vi "MEDIDA-IV-BK-8502-ELOAD.vi"() -> ()   [LabVIEW 2013]
doc: "This example shows how to configure a measurement and take multiple readings."
uses:
  <vilib>/Utility/NIReport.llb/HTML Report Image Alignment.ctl
  <vilib>/Utility/NIReport.llb/NI_report.lvclass
  <instrlib>/Keithley 2100 Series/Public/Configure/Configure DC Volts.vi
  <vilib>/Utility/file.llb/Write To Spreadsheet File (DBL).vi
  <vilib>/Utility/NIReport.llb/Append Report Text (str wrap).vi
  <vilib>/Analysis/NI_AALPro.lvlib
  <vilib>/Utility/NIReport.llb/NI_ReportGenerationCore.lvlib
  <instrlib>/Keithley 2100 Series/Keithley 2100 Series.lvlib
  <instrlib>/BK Precision 85XX Series/BK Precision 85XX Series.lvlib
  <instrlib>/Keithley 2100 Series/Public/Configure/Configure AC Volts.vi
  <instrlib>/Keithley 2100 Series/Public/Configure/Configure DC Current.vi
  <instrlib>/Keithley 2100 Series/Public/Configure/Configure 2 Wire Resistance.vi
  <instrlib>/Keithley 2100 Series/Public/Configure/Configure 4 Wire Resistance.vi
  <instrlib>/Keithley 2100 Series/Public/Configure/Configure AC Current.vi
panel:
  in  "Serial Configuration":T1={"Baud Rate"=9600, "Parity"=0, "Data Bits"=8, "Stop Bits"=10} {"Stop Bits" items=["1.0"=10]; "Data Bits" items=["8"=8]; "Parity" items=["None", "Odd", "Even"]; "Baud Rate" items=["4800"=4800, "9600"=9600, "19200"=19200, "38400"=38400]}
  in  "Tab Control 2":enum32{"Page 0", "Page 1", "Page 2"}(tab)
  out "?":dbl[](graph)
  in  "Digital Filter Readings (10)":i32=10
  in  "Digital Filter (0: Off)":u16(ring) items=["Off", "Moving Filter", "Repeating Filter"]
  in  "Delay Time (s)":dbl=1.0
  in  "Salvar em":path
  in  "stop":bool
  out "?":dbl[](graph)
  out "Voltage":dbl
  out "Curva I(V)":cluster{"Y":dbl[], "Y":dbl[]}[](graph)
  out "Fit linear R (Ohms)":dbl format="%#_4p"
  out "Current":dbl format="%#_6e"
  out "Temperatura (ºC)":dbl(slide) scale=0.0..100.0
  in  "Nº de células":dbl=1.0 format="%#.2g"
  out "Efficiency (%)":dbl
  out "Imp (Amps)":dbl
  out "Vmp (Volts)":dbl
  out "Pmax (Watts)":dbl
  out "Rshunt (Ohms)":dbl format="%.5f"
  out "Rseries (Ohms)":dbl format="%.5f"
  out "Fill Factor":dbl format="%.5f"
  out "Voc (Volts)":dbl format="%.5f"
  out "Isc (Amps)":dbl format="%.5f"
  in  "Área total das células (m²)":dbl=0.000988
  out "Luminosidade (W/m²)":dbl(knob) scale=0.0..1500.0
  out "Current and Power vs. Voltage":cluster{"voltage":dbl[], "current":dbl[]}[](graph)=[{"voltage"=[0.00134, 0.011411, 0.025834, 0.043904, 0.055853, 0.075347, 0.099155, 0.125663, 0.165263, 0.217428, 0.267874, 0.315752, 0.36725, 0.425099, 0.474937, 0.530085, 0.588472, 0.643221, 0.694358, 0.754622, 0.812053, 0.873564, 0.938448, 0.995444, 1.055319, 1.116484, 1.181096, 1.242979, 1.310054, 1.384923, 1.457974, 1.528483, 1.591961, 1.655914, 1.723383, 1.78537, 1.841803, 1.874735, 1.918172, 1.968127, 2.017264, 2.064175, 2.116398, 2.158177, 2.191225, 2.218755, 2.24048, 2.261856, 2.280808, 2.297463, 2.312474, 2.325391, 2.338537, 2.350645, 2.362017, 2.372641, 2.381227, 2.390448, 2.39921, 2.407016, 2.414358, 2.421423, 2.428593, 2.435115, 2.441853, 2.447216, 2.45325, 2.459011, 2.464522, 2.470157, 2.474042, 2.47733, 2.481663, 2.486527, 2.491175, 2.496801, 2.501739, 2.507229, 2.511954, 2.515881, 2.519776, 2.523798, 2.526966, 2.530482, 2.534179, 2.537454, 2.540996, 2.544249, 2.547457, 2.550411, 2.553712, 2.556938, 2.559943, 2.562754, 2.565624, 2.568656, 2.571368, 2.573971, 2.576844, 2.579394, 2.581922, 2.584569, 2.58696, 2.589667, 2.592003, 2.594428, 2.596938, 2.59895, 2.601485, 2.603775, 2.606028, 2.608198, 2.610307, 2.6125, 2.614489, 2.616517, 2.618693, 2.620546, 2.622788, 2.624713, 2.626775, 2.628652, 2.630374, 2.632358, 2.634291, 2.635909, 2.637872, 2.639706, 2.6416, 2.64327, 2.64507, 2.646937, 2.64855, 2.650292, 2.651969, 2.653556, 2.655158, 2.656701, 2.658523, 2.66009, 2.661507, 2.663332, 2.664731, 2.666314, 2.667904, 2.669272, 2.67096, 2.672271, 2.67381, 2.675234, 2.676598, 2.67819, 2.679489, 2.681023, 2.682384, 2.683646, 2.68527, 2.686444, 2.688037, 2.689359, 2.69057, 2.692017, 2.693188, 2.694379, 2.695854, 2.697093, 2.698419, 2.699635, 2.700981, 2.702147, 2.703366, 2.704606, 2.705739, 2.707068, 2.708254, 2.70947, 2.710647, 2.711858, 2.713057, 2.714301, 2.71546, 2.716741, 2.717737, 2.719024, 2.720152, 2.72107, 2.722252, 2.723341, 2.724516, 2.725631, 2.726557, 2.727808, 2.728738, 2.72989, 2.731069, 2.732, 2.733089, 2.734104, 2.73519, 2.736257, 2.737217, 2.738296, 2.739307, 2.740423, 2.741454, 2.742348, 2.743357, 2.744268, 2.745417, 2.746408, 2.747273, 2.74838, 2.749326, 2.750382, 2.751351, 2.752211, 2.753257, 2.754209, 2.755152, 2.756018, 2.756854, 2.757837, 2.758826, 2.759727, 2.760683, 2.761421, 2.76238, 2.763236, 2.764109, 2.764945, 2.76579, 2.76688, 2.767667, 2.768646, 2.769522, 2.770365, 2.771362, 2.772145, 2.773009, 2.7739, 2.774781, 2.775641, 2.776447, 2.777355, 2.778196, 2.778952, 2.779808], "current"=[0.11683, 0.116793, 0.116696, 0.116612, 0.116353, 0.116156, 0.115983, 0.115806, 0.115674, 0.115608, 0.115475, 0.115277, 0.115048, 0.114847, 0.114559, 0.114304, 0.114054, 0.113759, 0.113435, 0.11314, 0.112824, 0.112487, 0.112162, 0.111794, 0.111412, 0.111022, 0.11061, 0.110173, 0.109698, 0.109199, 0.108699, 0.1082, 0.107699, 0.107197, 0.106697, 0.106198, 0.105698, 0.105198, 0.104695, 0.104194, 0.103695, 0.103195, 0.102695, 0.102193, 0.101693, 0.101194, 0.100694, 0.10019, 0.09969, 0.09919, 0.098688, 0.098188, 0.097687, 0.097188, 0.096685, 0.096185, 0.095685, 0.095182, 0.094683, 0.094182, 0.093684, 0.093181, 0.092681, 0.09218, 0.091678, 0.091179, 0.090679, 0.090175, 0.089677, 0.089173, 0.088675, 0.088175, 0.087671, 0.087173, 0.086673, 0.086171, 0.085671, 0.085168, 0.08467, 0.08417, 0.083668, 0.083169, 0.082665, 0.082166, 0.081662, 0.081164, 0.080665, 0.080162, 0.079663, 0.079161, 0.07866, 0.078158, 0.077659, 0.077157, 0.076657, 0.076154, 0.075655, 0.075152, 0.074654, 0.074151, 0.073652, 0.07315, 0.07265, 0.072148, 0.071649, 0.071146, 0.070648, 0.070145, 0.069642, 0.069142, 0.068641, 0.068141, 0.067638, 0.067141, 0.066638, 0.066136, 0.065636, 0.065134, 0.064635, 0.064133, 0.063635, 0.063132, 0.062629, 0.06213, 0.061629, 0.061126, 0.060626, 0.060125, 0.059626, 0.059125, 0.058622, 0.058124, 0.057621, 0.057119, 0.056621, 0.056118, 0.055616, 0.055117, 0.054616, 0.054112, 0.053614, 0.053113, 0.05261, 0.052112, 0.051611, 0.051108, 0.05061, 0.050108, 0.049607, 0.049108, 0.048606, 0.048102, 0.047606, 0.047103, 0.046601, 0.046103, 0.045601, 0.045099, 0.044597, 0.044099, 0.043596, 0.043094, 0.042597, 0.042095, 0.041591, 0.041095, 0.040592, 0.040089, 0.039591, 0.03909, 0.038588, 0.038087, 0.037589, 0.037087, 0.036585, 0.036086, 0.035586, 0.035083, 0.034584, 0.034083, 0.033583, 0.033083, 0.032581, 0.03208, 0.031582, 0.03108, 0.030583, 0.030082, 0.029579, 0.02908, 0.02858, 0.028078, 0.02758, 0.02708, 0.026582, 0.026079, 0.025578, 0.025081, 0.02458, 0.02408, 0.02358, 0.023082, 0.02258, 0.022079, 0.021581, 0.021081, 0.020581, 0.020081, 0.019536, 0.019036, 0.018535, 0.018034, 0.017533, 0.017033, 0.016532, 0.016031, 0.01553, 0.01503, 0.014529, 0.014028, 0.013528, 0.013027, 0.012526, 0.012026, 0.011525, 0.011024, 0.010524, 0.010023, 0.009523, 0.009022, 0.008521, 0.00802, 0.007519, 0.007018, 0.006517, 0.006016, 0.005515, 0.005015, 0.004514, 0.004013, 0.003512, 0.003012, 0.002512, 0.002012, 0.001507, 0.001006, 0.000505]}, {"voltage"=[0.00134, 0.011411, 0.025834, 0.043904, 0.055853, 0.075347, 0.099155, 0.125663, 0.165263, 0.217428, 0.267874, 0.315752, 0.36725, 0.425099, 0.474937, 0.530085, 0.588472, 0.643221, 0.694358, 0.754622, 0.812053, 0.873564, 0.938448, 0.995444, 1.055319, 1.116484, 1.181096, 1.242979, 1.310054, 1.384923, 1.457974, 1.528483, 1.591961, 1.655914, 1.723383, 1.78537, 1.841803, 1.874735, 1.918172, 1.968127, 2.017264, 2.064175, 2.116398, 2.158177, 2.191225, 2.218755, 2.24048, 2.261856, 2.280808, 2.297463, 2.312474, 2.325391, 2.338537, 2.350645, 2.362017, 2.372641, 2.381227, 2.390448, 2.39921, 2.407016, 2.414358, 2.421423, 2.428593, 2.435115, 2.441853, 2.447216, 2.45325, 2.459011, 2.464522, 2.470157, 2.474042, 2.47733, 2.481663, 2.486527, 2.491175, 2.496801, 2.501739, 2.507229, 2.511954, 2.515881, 2.519776, 2.523798, 2.526966, 2.530482, 2.534179, 2.537454, 2.540996, 2.544249, 2.547457, 2.550411, 2.553712, 2.556938, 2.559943, 2.562754, 2.565624, 2.568656, 2.571368, 2.573971, 2.576844, 2.579394, 2.581922, 2.584569, 2.58696, 2.589667, 2.592003, 2.594428, 2.596938, 2.59895, 2.601485, 2.603775, 2.606028, 2.608198, 2.610307, 2.6125, 2.614489, 2.616517, 2.618693, 2.620546, 2.622788, 2.624713, 2.626775, 2.628652, 2.630374, 2.632358, 2.634291, 2.635909, 2.637872, 2.639706, 2.6416, 2.64327, 2.64507, 2.646937, 2.64855, 2.650292, 2.651969, 2.653556, 2.655158, 2.656701, 2.658523, 2.66009, 2.661507, 2.663332, 2.664731, 2.666314, 2.667904, 2.669272, 2.67096, 2.672271, 2.67381, 2.675234, 2.676598, 2.67819, 2.679489, 2.681023, 2.682384, 2.683646, 2.68527, 2.686444, 2.688037, 2.689359, 2.69057, 2.692017, 2.693188, 2.694379, 2.695854, 2.697093, 2.698419, 2.699635, 2.700981, 2.702147, 2.703366, 2.704606, 2.705739, 2.707068, 2.708254, 2.70947, 2.710647, 2.711858, 2.713057, 2.714301, 2.71546, 2.716741, 2.717737, 2.719024, 2.720152, 2.72107, 2.722252, 2.723341, 2.724516, 2.725631, 2.726557, 2.727808, 2.728738, 2.72989, 2.731069, 2.732, 2.733089, 2.734104, 2.73519, 2.736257, 2.737217, 2.738296, 2.739307, 2.740423, 2.741454, 2.742348, 2.743357, 2.744268, 2.745417, 2.746408, 2.747273, 2.74838, 2.749326, 2.750382, 2.751351, 2.752211, 2.753257, 2.754209, 2.755152, 2.756018, 2.756854, 2.757837, 2.758826, 2.759727, 2.760683, 2.761421, 2.76238, 2.763236, 2.764109, 2.764945, 2.76579, 2.76688, 2.767667, 2.768646, 2.769522, 2.770365, 2.771362, 2.772145, 2.773009, 2.7739, 2.774781, 2.775641, 2.776447, 2.777355, 2.778196, 2.778952, 2.779808], "current"=[0.0001565522, 0.0013327249229999998, 0.0030147244639999998, 0.0051197332479999995, 0.0064986641089999995, 0.008752006132, 0.011500294365, 0.014552529378000001, 0.019116632262, 0.025136416224, 0.030932750149999997, 0.036398943304, 0.042251378, 0.048821344853, 0.054408307782999994, 0.06059083584, 0.067117585488, 0.073172177739, 0.07876449972999999, 0.08537793308000001, 0.091619067672, 0.098264593668, 0.10525820457599999, 0.111284666536, 0.11757520042799999, 0.123954286648, 0.13064102855999998, 0.136942725367, 0.14371030369200002, 0.151232206677, 0.15848031582600003, 0.1653818606, 0.171452607739, 0.17750901305800001, 0.183879795951, 0.18960272326, 0.194674893494, 0.19721837253, 0.20082301753999998, 0.20506702463799997, 0.20918019047999997, 0.213012539125, 0.21734349260999997, 0.220550582161, 0.22283224392500003, 0.22452469346999998, 0.22560289311999998, 0.22661535264, 0.22737374952, 0.22788535497, 0.22821343411199999, 0.22832549150800002, 0.228444663919, 0.22845448626, 0.22837161364499997, 0.228212474585, 0.22784770549500002, 0.227527621536, 0.22716440043000002, 0.226697580912, 0.226186714872, 0.22563061656299999, 0.22508442783299998, 0.2244689007, 0.22386419933399998, 0.223134707664, 0.22245825675, 0.221741316925, 0.22101093939400002, 0.220271310161, 0.21938567435, 0.21843857275, 0.217569876873, 0.21675801817100002, 0.21591761077500002, 0.215151838971, 0.214326481869, 0.213535679472, 0.21268714517999998, 0.21176170376999998, 0.210824618368, 0.20990175586200002, 0.20889164439, 0.20791958401200003, 0.20694612549799998, 0.205949916456, 0.20496944233999997, 0.20395208833800002, 0.202938066991, 0.201893085171, 0.20087498591999997, 0.19984516020400003, 0.198802613437, 0.19773441037800002, 0.196673038968, 0.19561342902399997, 0.19453684604000002, 0.19343906859199997, 0.19237171197599998, 0.191264644494, 0.190163719144, 0.18906122235000003, 0.18794264400000002, 0.186839294716, 0.18571442294700002, 0.18458317448800002, 0.18346847582400003, 0.18230334774999998, 0.18117261836999998, 0.18003021105, 0.17888036794799997, 0.17772521991799997, 0.17655594486600001, 0.1754058625, 0.174224317982, 0.173045968312, 0.171880533748, 0.170686643164, 0.16952390237999998, 0.16833071882899997, 0.167154827125, 0.16595205806399999, 0.16473769324600002, 0.16354840254, 0.16234872003900003, 0.161122573534, 0.159923627872, 0.15871232324999998, 0.15750804159999998, 0.15628333874999997, 0.15505929354, 0.153850566188, 0.15261209955000002, 0.151382028748, 0.15015713674899997, 0.148912255608, 0.147669267328, 0.146429389017, 0.145197892168, 0.14394279008, 0.142694036298, 0.141457552516, 0.14019149791, 0.13894695516799999, 0.137693193344, 0.136421153376, 0.1351772856, 0.13390215526799998, 0.13263969267, 0.131375391272, 0.130098722388, 0.12882629537999998, 0.127559753334, 0.126284226369, 0.12500177678399998, 0.12372413153799999, 0.12245099727000001, 0.12115593795599999, 0.11987838608899999, 0.118598042541, 0.11729808972000001, 0.11600978059799999, 0.11472172923600002, 0.113419884005, 0.11212326371400001, 0.110837036835, 0.109534224048, 0.10822566751499998, 0.10693453877100001, 0.10562692623, 0.10431748720799999, 0.10301032872200001, 0.10170602327099999, 0.10039703091600001, 0.09908147259000001, 0.09777393442, 0.096461084142, 0.09514011421400001, 0.093828363288, 0.092511520983, 0.09119329318000001, 0.089877942503, 0.088546589197, 0.08722628991999999, 0.085907840464, 0.08457085560000001, 0.08325463291600001, 0.08192354396200001, 0.080588458764, 0.07926134948, 0.07792499906000001, 0.07659139302399999, 0.07525859404, 0.07392542120000001, 0.072597276158, 0.07124782800000001, 0.069906950442, 0.06857406242399999, 0.0672309702, 0.06588906856, 0.06454357686, 0.063205348272, 0.061853552060000004, 0.060505799417, 0.059163318774, 0.05781143818799999, 0.056461030417, 0.055107645708, 0.05363446651200001, 0.052280622688, 0.050920705054999994, 0.04956428492000001, 0.048203932758, 0.046847256606, 0.045485334732000005, 0.044120694541, 0.04275808121, 0.04139576127, 0.040029603408, 0.038661420504, 0.037294720912, 0.035926342599, 0.034557054476, 0.033188476902, 0.031816871575, 0.030441905104, 0.02907128712, 0.027695914428000002, 0.026322610007, 0.024945333790000003, 0.02356729659, 0.0221903776, 0.020810088172999997, 0.019430357627999998, 0.018048974874, 0.01666651584, 0.015284061429999999, 0.013902307175000002, 0.012517362625999999, 0.011131660699999999, 0.009745030872, 0.008360230691999999, 0.006974434864, 0.00558803826, 0.004186741372, 0.0027956257119999997, 0.0014038030400000002]}]
  in  "Tab Control":enum32{"INICIAL", "CONFIG"}(tab)=enum."CONFIG"
  in  "BK 8500":refnum<visa-resource-name>="GPIB0::24::INSTR"
  in  "Keithley 2100 Pyranometer":refnum<visa-resource-name>="GPIB::16"
  in  "Keithley 2100 PT100":refnum<visa-resource-name>="GPIB::16"
  in  "Monitorar?":bool
  in  "Multimetro p/ V":refnum<visa-resource-name>
  in  "Salvar Medidas em":path
  in  "Fonte Inicial (V ou A)":dbl format="%.3e"
  in  "Fonte Final (V ou A)":dbl format="%.3e"
  in  "Passo Fonte (V ou A)":dbl format="%.3e"
  in  "Salvar relatório em":path
  in  "Maximum Input Voltage (0)":dbl min=0.0 max=120.0 format="%#_3g"
  in  "Maximum Input Current (0)":dbl min=0.0 max=30.0 format="%#_3g"
  in  "Maximum Input Power (0)":dbl min=0.0 max=300.0 step=1.0 format="%#_3g"
  # "Programa desenvolvido \nem plataforma LABVIEW 2010:\n2017\nLSD/UNIFEI\nRero e Davi"
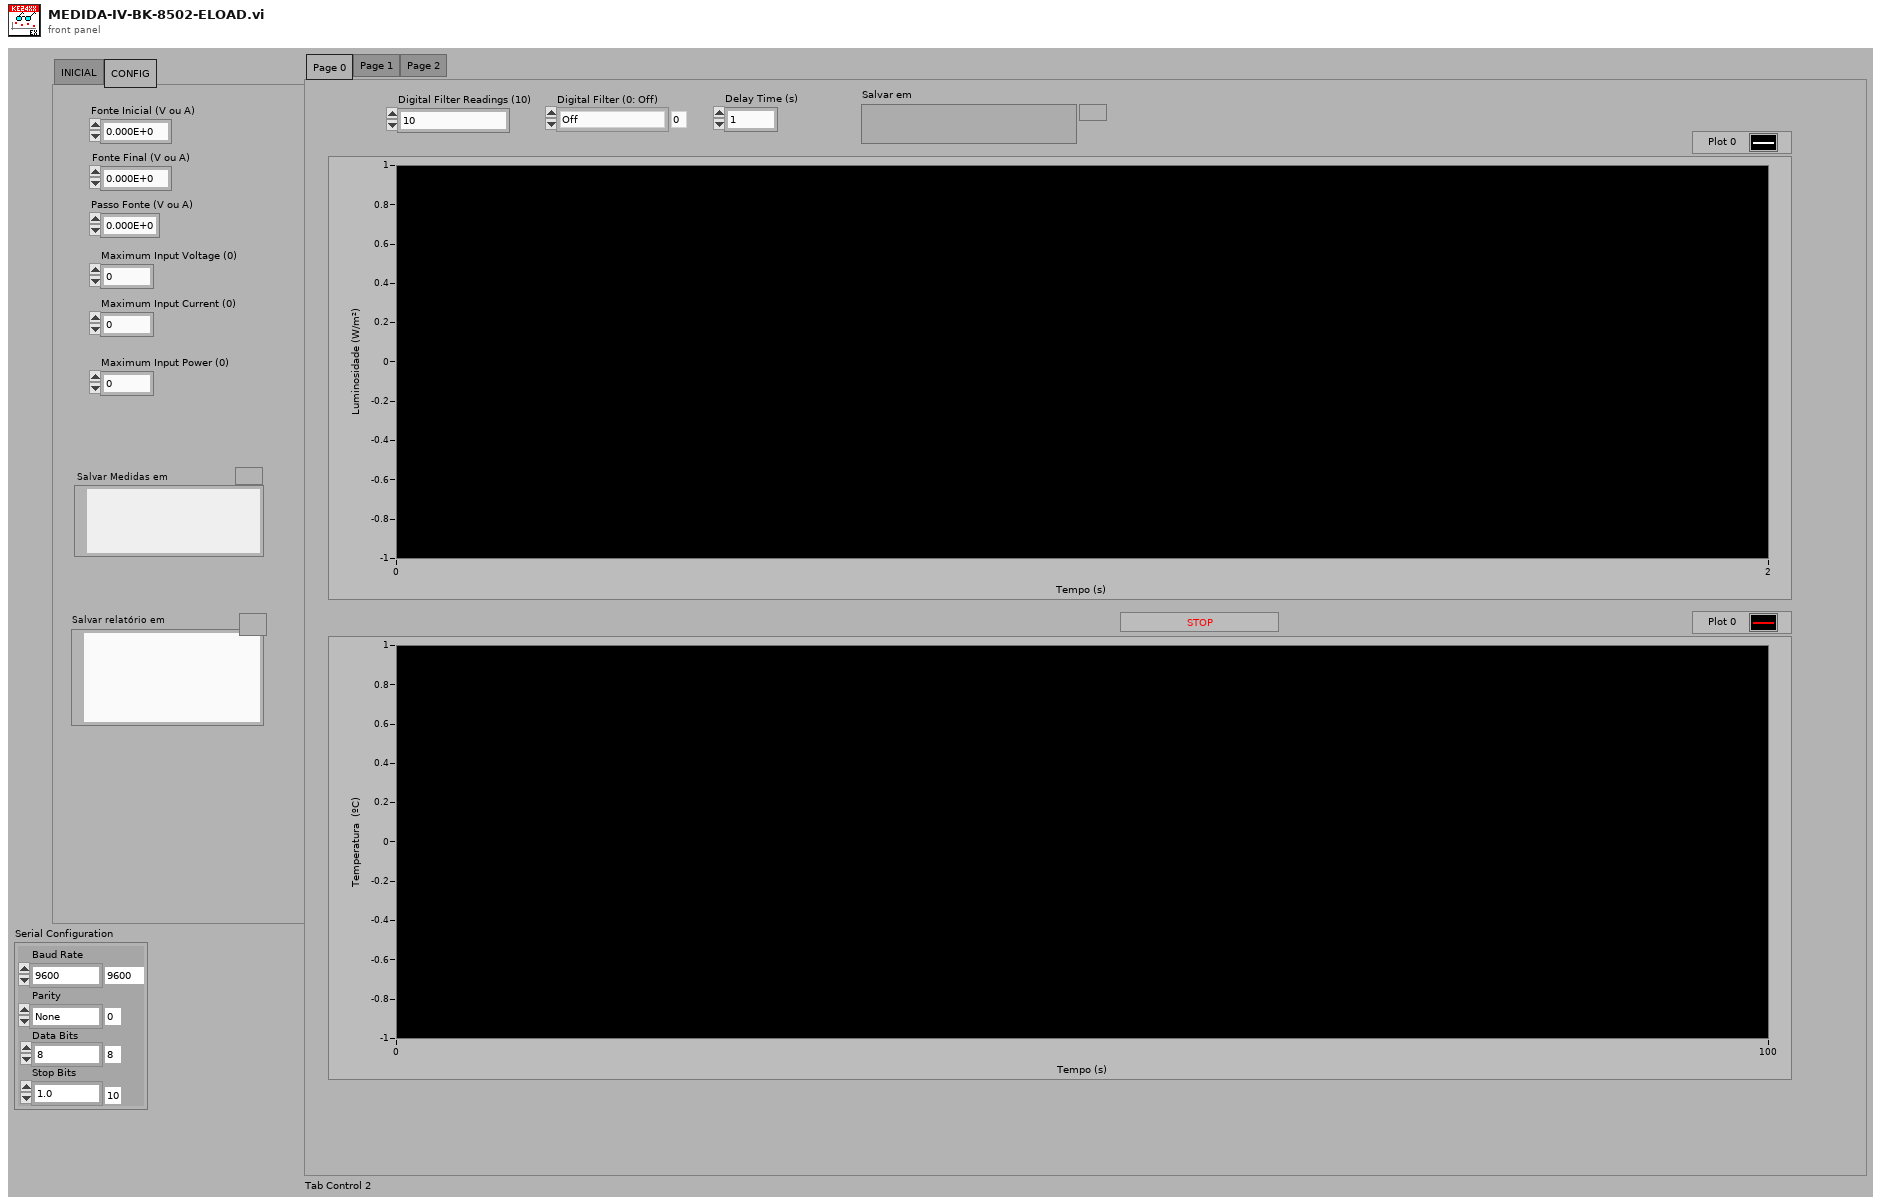
[diagram p1: front panel]
types:
  T1 = cluster{"Baud Rate":u32, "Parity":u16, "Data Bits":u16, "Stop Bits":u16}
  T2 = typedef "NI_ReportGenerationCore.lvlib/HTML Report Image Alignment.ctl" = enum16{"(default)", "LEFT", "RIGHT", "TOP", "TEXTTOP", "MIDDLE", "ABSMIDDLE", "BASELINE", "BOTTOM", "ABSBOTTOM"}
  T3 = cluster{"Italic":enum16{"Italic Unchanged", "Italic On", "Italic Off"}, "Strike Through":enum16{"Strike Through Unchanged", "Strike Through On", "Strike Through Off"}, "Underline":enum16{"Underline Unchanged", "Underline On", "Underline Off"}, "Bold":enum16{"Bold Unchanged", "Bold On", "Bold Off"}}
  T4 = enum16{"Standard Report", "HTML", "Word", "Excel"}
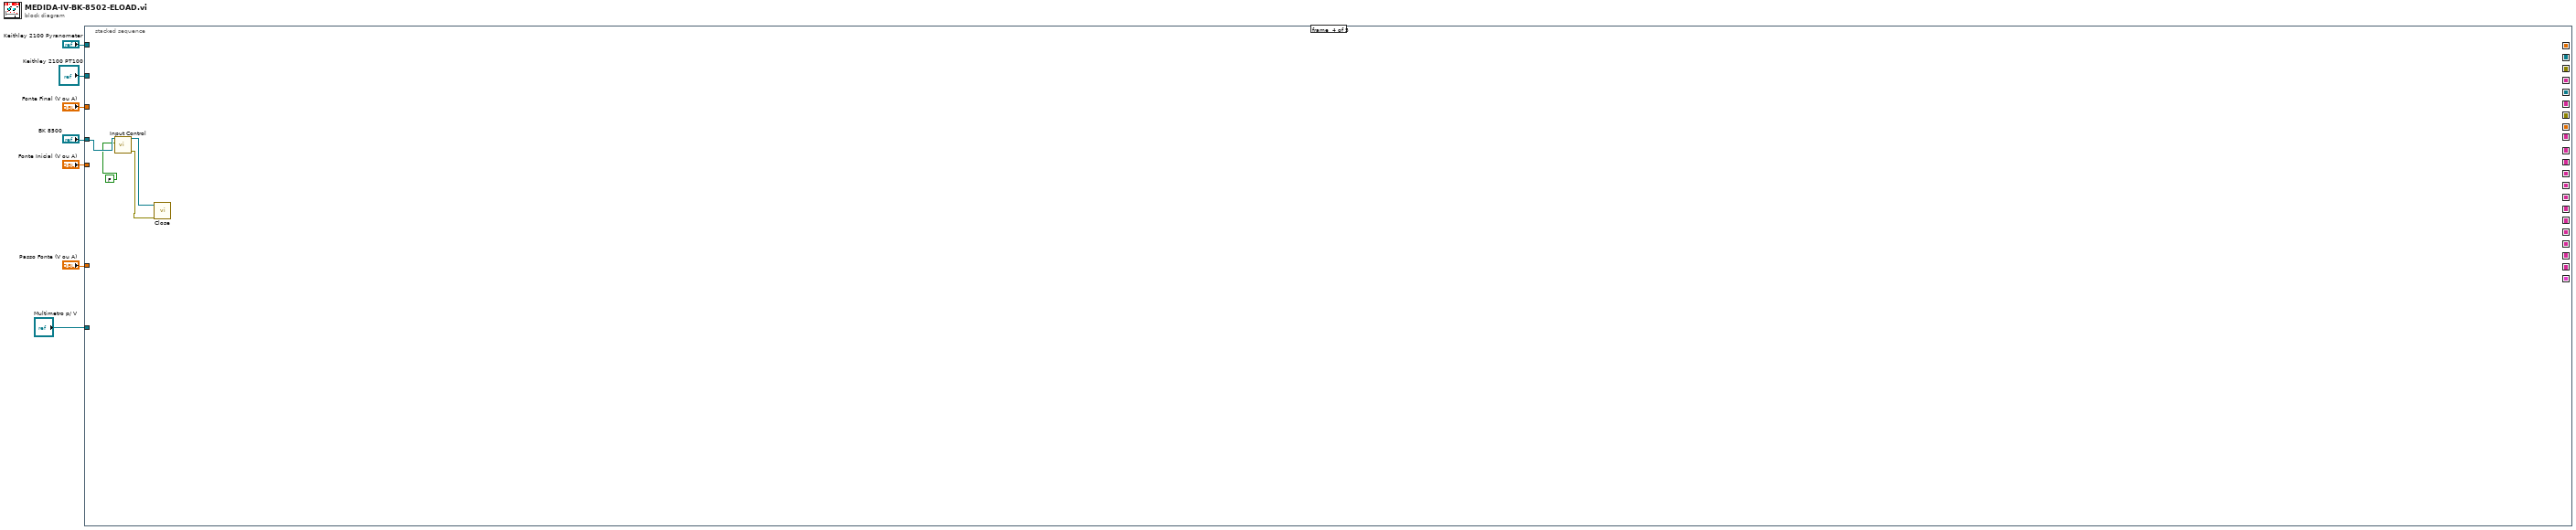
[diagram p0: block diagram]
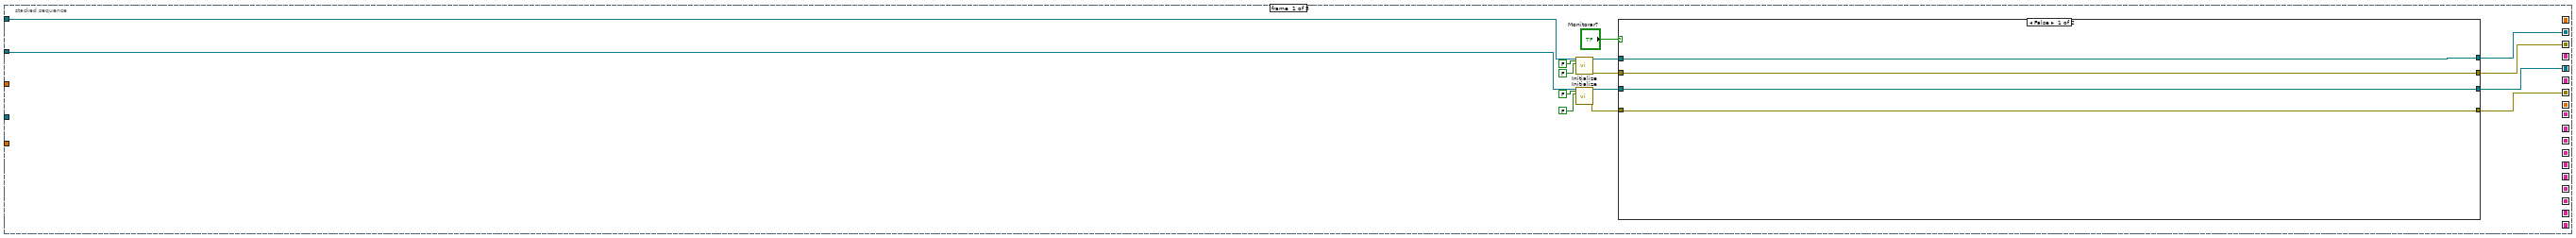
[diagram p2: hidden frame]
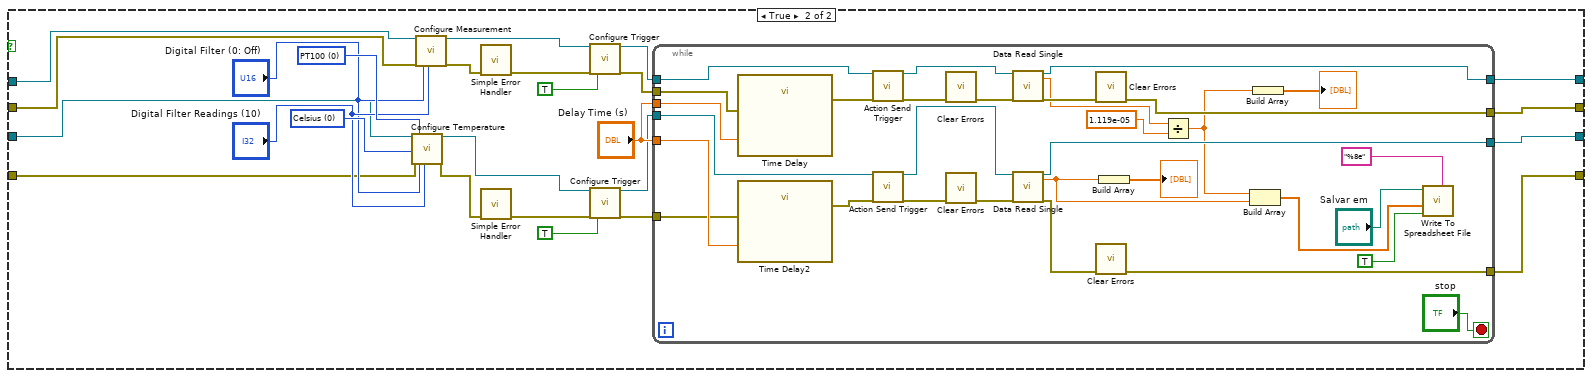
[diagram p3: hidden frame]
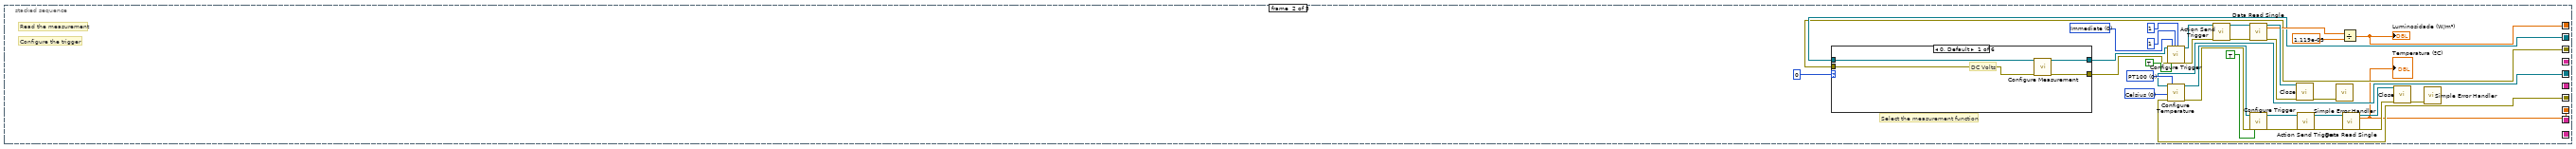
[diagram p4: hidden frame]
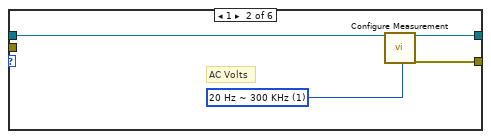
[diagram p5: hidden frame]
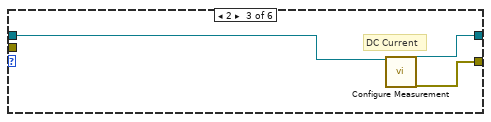
[diagram p6: hidden frame]
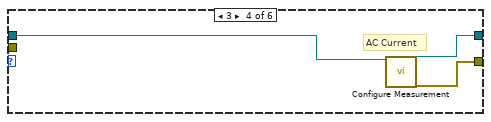
[diagram p7: hidden frame]
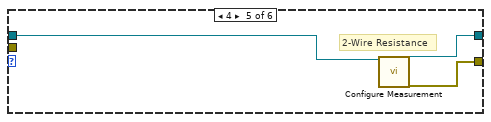
[diagram p8: hidden frame]
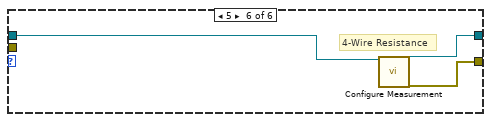
[diagram p9: hidden frame]
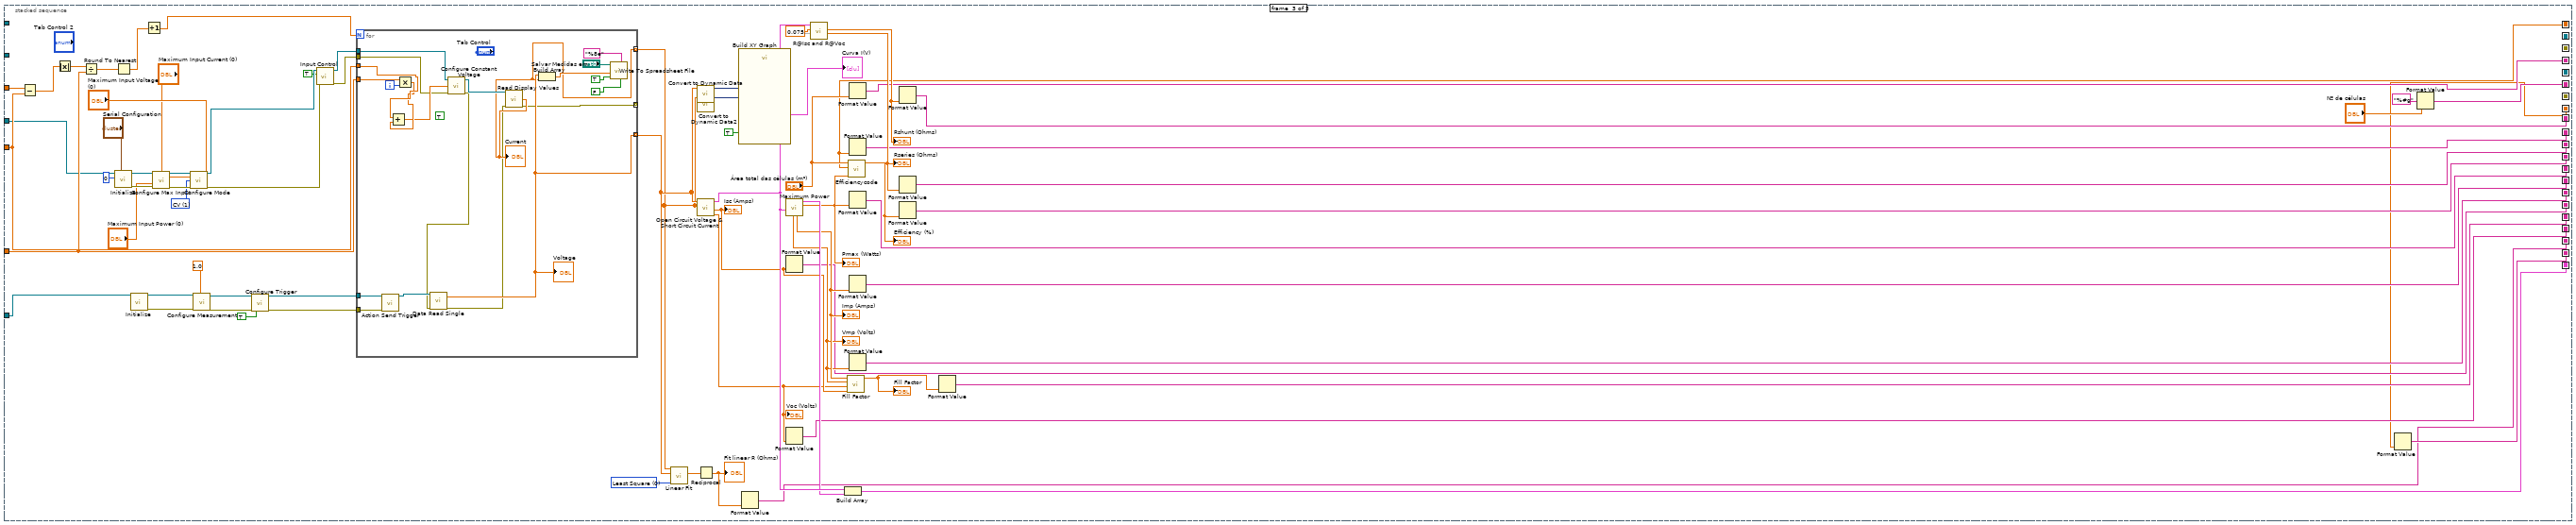
[diagram p10: hidden frame]
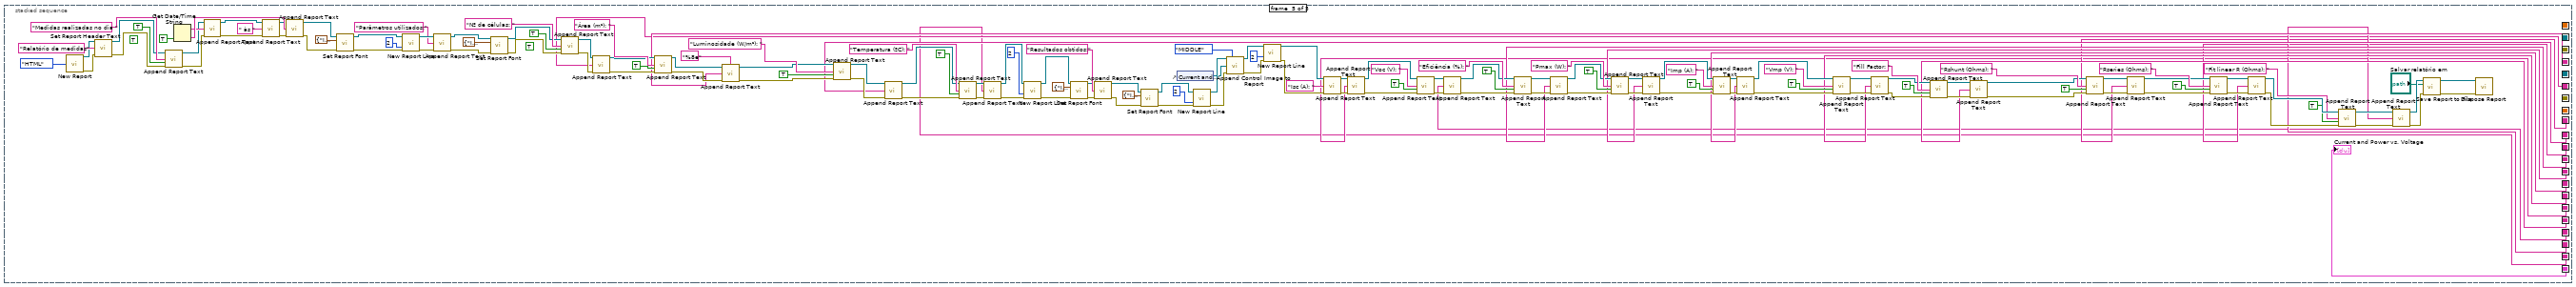
[diagram p11: hidden frame]
diagram:
  n1 = stacked-sequence {
    seq-local: [_ w100 _ _ _] -> [_ _ w180 _ _]
    seq-local: [_ _ w179 _ _] -> [_ _ _ _ w239]
    seq-local: [_ _ w178 _ _] -> [_ _ _ _ w240]
    seq-local: [_ _ w177 _ _] -> [_ _ _ _ w241]
    seq-local: [_ _ w176 _ _] -> [_ _ _ _ w242]
    seq-local: [_ _ w175 _ _] -> [_ _ _ _ w243]
    seq-local: [_ _ w174 _ _] -> [_ _ _ _ w244]
    seq-local: [_ _ w173 _ _] -> [_ _ _ _ w246]
    seq-local: [_ _ w172 _ _] -> [_ _ _ _ w247]
    seq-local: [_ _ w171 _ _] -> [_ _ _ _ w248]
    seq-local: [_ _ w170 _ _] -> [_ _ _ _ w249]
    seq-local: [_ _ w169 _ _] -> [_ _ _ _ w250]
    seq-local: [_ _ w168 _ _] -> [_ _ _ _ w251]
    seq-local: [_ _ w167 _ _] -> [_ _ _ _ w252]
    seq-local: [_ _ w166 _ _] -> [_ _ _ _ w245]
    seq-local: [_ _ w165 _ _] -> [_ _ _ _ w238]
    seq-local: [_ w83 _ _ _] -> [_ _ w163 _ _]
    seq-local: [w19 _ _ _ _] -> [_ w93 _ _ _]
    seq-local: [w20 _ _ _ _] -> [_ w94 _ _ _]
    seq-local: [w18 _ _ _ _] -> [_ w92 _ _ _]
    seq-local: [w17 _ _ _ _] -> [_ w91 _ _ _]
    tunnel: "BK 8500" -> [_ _ w152 w235 _]
    tunnel: "Fonte Inicial (V ou A)" -> [_ _ w205 _ _]
    tunnel: "Fonte Final (V ou A)" -> [_ _ w204 _ _]
    tunnel: "Passo Fonte (V ou A)" -> [_ _ w203 _ _]
    tunnel: "Keithley 2100 Pyranometer" -> [w22 _ _ _ _]
    tunnel: "Keithley 2100 PT100" -> [w21 _ _ _ _]
    tunnel: "Multimetro p/ V" -> [_ _ w155 _ _]
    frame #0 {
      n2 = call <instrlib>:"Initialize.vi"("VISA resource name"=w22, "ID Query? (T: Check)"=FALSE, "Reset? (T: Reset)"=FALSE) -> ("VISA resource name out"=w10:refnum<visa-resource-name>, "error out"=w9:errorcluster)  [unwired: 15 in]
      n3 = call <instrlib>:"Initialize.vi"("VISA resource name"=w21, "ID Query? (T: Check)"=FALSE, "Reset? (T: Reset)"=FALSE) -> ("VISA resource name out"=w12:refnum<visa-resource-name>, "error out"=w11:errorcluster)  [unwired: 15 in]
      n4 = case shown="False" "Monitorar?" {
        tunnel: [w26 w44] -> w20
        tunnel: [w24 w28] -> w19
        tunnel: [w25 w43] -> w18
        tunnel: [w23 w27] -> w17
        tunnel: w12 -> [w24 w35]
        tunnel: w11 -> [w23 w34]
        tunnel: w10 -> [w26 w33]
        tunnel: w9 -> [w25 w32]
        frame False {
        }
        frame True {
          w38 = u16 0 items=["PT100", "D100", "F100", "PT385", "PT3916", "User-Defined", "SPRTD", "NTCT"] ("RTD Type  (PT100)")
          w47 = u16 0 items=["Celsius", "Fahrenheit", "Kelvin"] ("Temperature Units (0: Celsius)")
          n5 = call <instrlib>:"Configure Temperature.vi"("VISA resource name"=w35, "Temperature Units (0: Celsius)"=w47, "error in (no error)"=w34, "RTD Type  (PT100)"=w38, "Digital Filter (0: Off)"="Digital Filter (0: Off)", "Digital Filter Readings (10)"="Digital Filter Readings (10)") -> ("VISA resource name out"=w46:refnum<visa-resource-name>, "error out"=w40:errorcluster)  [unwired: 12 in]
          n6 = call-poly <instrlib>:"Configure Measurement.vi"("VISA resource name"=w33, "error in (no error)"=w32, "Digital Filter (0: Off)"="Digital Filter (0: Off)", "Digital Filter Readings (10)"="Digital Filter Readings (10)") -> ("VISA resource name out"=w50:refnum<visa-resource-name>, "error out"=w42:errorcluster)  [unwired: 14 in]
          n7 = call <vilib>:"Simple Error Handler.vi"("error in (no error)"=w42) -> ("error out"=w41:errorcluster)  [unwired: 4 in, 4 out]
          n8 = call <vilib>:"Simple Error Handler.vi"("error in (no error)"=w40) -> ("error out"=w39:errorcluster)  [unwired: 4 in, 4 out]
          n9 = call <instrlib>:"Configure Trigger.vi"("VISA resource name"=w50, "error in (no error)"=w41, "Auto Delay? (T: Auto)"=TRUE) -> ("VISA resource name out"=w48:refnum<visa-resource-name>, "error out"=w49:errorcluster)  [unwired: 15 in]
          n10 = call <instrlib>:"Configure Trigger.vi"("VISA resource name"=w46, "error in (no error)"=w39, "Auto Delay? (T: Auto)"=TRUE) -> ("VISA resource name out"=w30:refnum<visa-resource-name>, "error out"=w29:errorcluster)  [unwired: 15 in]
          n11 = while {
            tunnel: w49 -> [w80]
            tunnel: "Delay Time (s)" -> [w79]
            tunnel: w48 -> [w77]
            tunnel: [w70] -> w43
            tunnel: [w73] -> w44
            tunnel: "Delay Time (s)" -> [w60]
            tunnel: w30 -> [w59]
            tunnel: w29 -> [w58]
            tunnel: [w57] -> w28
            tunnel: [w56] -> w27
            stop <- "stop" stop-if-true
            n12 = call "Time Delay"("error in (no error)"=w80, "Delay Time (s)"=w79) -> ("error out"=w78:errorcluster)  [unwired: 9 in]
            n13 = call "Time Delay2"("error in (no error)"=w58, "Delay Time (s)"=w60) -> ("error out"=w66:errorcluster)  [unwired: 9 in]
            n14 = call <instrlib>:"Action Send Trigger.vi"("VISA resource name"=w77, "error in (no error)"=w78) -> ("VISA resource name out"=w82:refnum<visa-resource-name>, "error out"=w69:errorcluster)  [unwired: 16 in]
            n15 = call <instrlib>:"Action Send Trigger.vi"("VISA resource name"=w59, "error in (no error)"=w66) -> ("VISA resource name out"=w65:refnum<visa-resource-name>, "error out"=w64:errorcluster)  [unwired: 16 in]
            n16 = call <vilib>:"Clear Errors.vi"("error in (no error)"=w69) -> ("error out"=w68:errorcluster)  [unwired: 6 in]
            n17 = call <vilib>:"Clear Errors.vi"("error in (no error)"=w64) -> ("error out"=w63:errorcluster)  [unwired: 6 in]
            n18 = call <instrlib>:"Data Read Single.vi"("VISA resource name"=w82, "error in (no error)"=w68) -> ("VISA resource name out"=w73:refnum<visa-resource-name>, "Measurement"=w55:dbl, "error out"=w71:errorcluster)  [unwired: 15 in]
            n19 = call <instrlib>:"Data Read Single.vi"("VISA resource name"=w65, "error in (no error)"=w63) -> ("VISA resource name out"=w57:refnum<visa-resource-name>, "Measurement"=w53:dbl, "error out"=w62:errorcluster)  [unwired: 15 in]
            n20 = call <vilib>:"Clear Errors.vi"("error in (no error)"=w71) -> ("error out"=w70:errorcluster)  [unwired: 6 in]
            n21 = call <vilib>:"Clear Errors.vi"("error in (no error)"=w62) -> ("error out"=w56:errorcluster)  [unwired: 6 in]
            n22 = Build Array(w53) -> (→"?":dbl[])
            n23 = Divide(x=w55, y=1.119e-05) -> (x/y=w54:dbl)
            n24 = Build Array(w54, w53) -> (w52:dbl[])
            n25 = Build Array(w54) -> (→"?":dbl[])
            n26 = call-poly <vilib>:"Write To Spreadsheet File.vi"("format (%.3f)"="%8e", "append to file? (new file:F)"=TRUE, "1D data"=w52, "file path (dialog if empty)"="Salvar em") -> ()  [unwired: 4 in, 1 out]
          }
        }
      }
    }
    frame #1 {
      w95 = u16 0 items=["PT100", "D100", "F100", "PT385", "PT3916", "User-Defined", "SPRTD", "NTCT"] ("RTD Type  (PT100)")
      w96 = u16 0 items=["Celsius", "Fahrenheit", "Kelvin"] ("Temperature Units (0: Celsius)")
      w113 = u16 0 items=["Immediate", "Bus", "External"] ("Source (0: Immediate)")
      # "Read the measurement"
      # "Configure the trigger"
      # "Select the measurement function"
      n27 = case shown="0, Default" u16 0 ("Function (0: DC Volts)") {
        tunnel: w94 -> [w120 w124 w127 w130 w133 w136]
        tunnel: [w119 w123 w126 w129 w132 w135] -> w109
        tunnel: [w118 w122 w125 w128 w131 w134] -> w110
        tunnel: w92 -> [w117 _ _ _ _ _]
        frame 0, Default {
          # "DC Volts"
          n28 = call-poly <instrlib>:"Configure Measurement.vi"("VISA resource name"=w120, "error in (no error)"=w117) -> ("VISA resource name out"=w118:refnum<visa-resource-name>, "error out"=w119:errorcluster)  [unwired: 16 in]
        }
        frame 1 {
          w121 = u16 1 items=["3 Hz ~ 300 KHz", "20 Hz ~ 300 KHz", "200 Hz ~ 300 KHz"] ("Bandwidth (20 Hz)")
          # "AC Volts"
          n29 = call-poly <instrlib>:"Configure Measurement.vi"("VISA resource name"=w124, "Bandwidth (20 Hz)"=w121) -> ("VISA resource name out"=w122:refnum<visa-resource-name>, "error out"=w123:errorcluster)  [unwired: 16 in]
        }
        frame 2 {
          # "DC Current"
          n30 = call-poly <instrlib>:"Configure Measurement.vi"("VISA resource name"=w127) -> ("VISA resource name out"=w125:refnum<visa-resource-name>, "error out"=w126:errorcluster)  [unwired: 17 in]
        }
        frame 3 {
          # "AC Current"
          n31 = call-poly <instrlib>:"Configure Measurement.vi"("VISA resource name"=w130) -> ("VISA resource name out"=w128:refnum<visa-resource-name>, "error out"=w129:errorcluster)  [unwired: 17 in]
        }
        frame 4 {
          # "2-Wire Resistance"
          n32 = call-poly <instrlib>:"Configure Measurement.vi"("VISA resource name"=w133) -> ("VISA resource name out"=w131:refnum<visa-resource-name>, "error out"=w132:errorcluster)  [unwired: 17 in]
        }
        frame 5 {
          # "4-Wire Resistance"
          n33 = call-poly <instrlib>:"Configure Measurement.vi"("VISA resource name"=w136) -> ("VISA resource name out"=w134:refnum<visa-resource-name>, "error out"=w135:errorcluster)  [unwired: 17 in]
        }
      }
      n34 = call <instrlib>:"Configure Trigger.vi"("VISA resource name"=w110, "error in (no error)"=w109, "Source (0: Immediate)"=w113, "Auto Delay? (T: Auto)"=TRUE, "Sample Count (1)"=1, "Trigger Count (1)"=1) -> ("VISA resource name out"=w105:refnum<visa-resource-name>, "error out"=w104:errorcluster)  [unwired: 12 in]
      n35 = call <instrlib>:"Configure Temperature.vi"("VISA resource name"=w93, "Temperature Units (0: Celsius)"=w96, "error in (no error)"=w91, "RTD Type  (PT100)"=w95) -> ("VISA resource name out"=w90:refnum<visa-resource-name>, "error out"=w89:errorcluster)  [unwired: 14 in]
      n36 = call <instrlib>:"Action Send Trigger.vi"("VISA resource name"=w105, "error in (no error)"=w104) -> ("VISA resource name out"=w112:refnum<visa-resource-name>, "error out"=w111:errorcluster)  [unwired: 16 in]
      n37 = call <instrlib>:"Data Read Single.vi"("VISA resource name"=w112, "error in (no error)"=w111) -> ("VISA resource name out"=w107:refnum<visa-resource-name>, "Measurement"=w101:dbl, "error out"=w106:errorcluster)  [unwired: 15 in]
      n38 = call <instrlib>:"Configure Trigger.vi"("VISA resource name"=w90, "error in (no error)"=w89, "Auto Delay? (T: Auto)"=TRUE) -> ("VISA resource name out"=w87:refnum<visa-resource-name>, "error out"=w86:errorcluster)  [unwired: 15 in]
      n39 = call <instrlib>:"Close.vi"("VISA resource name"=w107, "error in (no error)"=w106) -> ("error out"=w108:errorcluster)  [unwired: 17 in]
      n40 = call <instrlib>:"Action Send Trigger.vi"("VISA resource name"=w87, "error in (no error)"=w86) -> ("VISA resource name out"=w85:refnum<visa-resource-name>, "error out"=w84:errorcluster)  [unwired: 16 in]
      n41 = call <vilib>:"Simple Error Handler.vi"("error in (no error)"=w108) -> ()  [unwired: 4 in, 5 out]
      n42 = Divide(x=w101, y=1.119e-05) -> (x/y=w100:dbl)
      "Luminosidade (W/m²)" <- w100
      n43 = call <instrlib>:"Data Read Single.vi"("VISA resource name"=w85, "error in (no error)"=w84) -> ("VISA resource name out"=w98:refnum<visa-resource-name>, "Measurement"=w83:dbl, "error out"=w97:errorcluster)  [unwired: 15 in]
      "Temperatura (ºC)" <- w83
      n44 = call <instrlib>:"Close.vi"("VISA resource name"=w98, "error in (no error)"=w97) -> ("error out"=w99:errorcluster)  [unwired: 17 in]
      n45 = call <vilib>:"Simple Error Handler.vi"("error in (no error)"=w99) -> ()  [unwired: 4 in, 5 out]
    }
    frame #2 {
      w145 = u16 1 items=["CC", "CV", "CW", "CR"] ("Mode of Operation (0:CC)")
      w198 = u16 0 items=["Least Square", "Least Absolute Residual", "Bisquare"] ("method")
      n46 = Subtract(x=w204, y=w205) -> (x-y=w210:dbl)
      n47 = Absolute Value(x=w210) -> (abs(x)=w209:dbl)
      n48 = Divide(x=w209, y=w203) -> (x/y=w208:dbl)
      n49 = call <instrlib>:"Initialize.vi"("Serial Configuration"="Serial Configuration", "Communication Address (0)"=u8 0, "VISA resource name"=w152) -> ("error out"=w148:errorcluster, "VISA resource name out"=w149:refnum<visa-resource-name>)  [unwired: 7 in]
      n50 = Round To Nearest(number=w208) -> (nearest integer value=w207:dbl)
      n51 = call <instrlib>:"Initialize.vi"("VISA resource name"=w155) -> ("VISA resource name out"=w154:refnum<visa-resource-name>, "error out"=w153:errorcluster)  [unwired: 17 in]
      n52 = Increment(x=w207) -> (x+1=w206:dbl)
      n53 = call <instrlib>:"Configure Max Input.vi"("VISA resource name"=w149, "Maximum Input Voltage (0)"="Maximum Input Voltage (0)", "Maximum Input Current (0)"="Maximum Input Current (0)", "Maximum Input Power (0)"="Maximum Input Power (0)", "error in (no error)"=w148) -> ("VISA resource name out"=w147:refnum<visa-resource-name>, "error out"=w146:errorcluster)  [unwired: 9 in]
      n54 = call <instrlib>:"Configure Mode.vi"("VISA resource name"=w147, "Mode of Operation (0:CC)"=w145, "error in (no error)"=w146) -> ("VISA resource name out"=w144:refnum<visa-resource-name>, "error out"=w139:errorcluster)  [unwired: 11 in]
      n55 = call-poly <instrlib>:"Configure Measurement.vi"("VISA resource name"=w154, "error in (no error)"=w153, "Custom Range (100mV)"=1.0) -> ("VISA resource name out"=w162:refnum<visa-resource-name>, "error out"=w161:errorcluster)  [unwired: 15 in]
      n56 = call <instrlib>:"Configure Trigger.vi"("VISA resource name"=w162, "error in (no error)"=w161, "Auto Delay? (T: Auto)"=TRUE) -> ("VISA resource name out"=w159:refnum<visa-resource-name>, "error out"=w158:errorcluster)  [unwired: 15 in]
      n57 = call <instrlib>:"Input Control.vi"("error in (no error)"=w139, "Enable Input Terminals (F: Off)"=TRUE, "VISA resource name"=w144) -> ("error out"=w138:errorcluster, "VISA resource name out"=w143:refnum<visa-resource-name>)  [unwired: 7 in]
      n58 = for {
        N: w206 -> [_]
        tunnel: w205 -> [w219]
        tunnel: w203 -> [w227]
        tunnel: [w221] -> w193 mode=indexing
        tunnel: [w215] -> w157 mode=indexing
        tunnel: w159 -> [w224]
        tunnel: w158 -> [w223]
        tunnel: [w211] -> _ mode=indexing
        tunnel: w143 -> [w220]
        tunnel: w138 -> [w214]
        i -> [w226]
        (unwired) TRUE ("Enable Output (T: Enable)")
        n59 = call <instrlib>:"Action Send Trigger.vi"("VISA resource name"=w224, "error in (no error)"=w223) -> ("VISA resource name out"=w222:refnum<visa-resource-name>)  [unwired: 16 in, 1 out]
        n60 = Multiply(x=w227, y=w226) -> (x*y=w218:dbl)
        n61 = Add(x=w219, y=w218) -> (x+y=w217:dbl)
        n62 = call <instrlib>:"Configure Constant Voltage.vi"("VISA resource name"=w220, "CV Voltage (0)"=w217, "error in (no error)"=w214) -> ("VISA resource name out"=w216:refnum<visa-resource-name>, "error out"=w213:errorcluster)  [unwired: 11 in]
        n63 = call <instrlib>:"Data Read Single.vi"("VISA resource name"=w222, "error in (no error)"=w213) -> ("Measurement"=w221:dbl, "error out"=w212:errorcluster)  [unwired: 15 in, 1 out]
        "Voltage" <- w221
        n64 = call <instrlib>:"Read Display Values.vi"("VISA resource name"=w216, "error in (no error)"=w212) -> ("Terminal Input Current (A)"=w215:dbl, "error out"=w211:errorcluster)  [unwired: 9 in, 3 out]
        "Current" <- w215
        n65 = Build Array(w221, w215) -> (w225:dbl[])
        n66 = call-poly <vilib>:"Write To Spreadsheet File.vi"("transpose? (no:F)"=FALSE ("append to file? (new file:F)"), "format (%.3f)"="%8e", "append to file? (new file:F)"=TRUE, "1D data"=w225, "file path (dialog if empty)"="Salvar Medidas em") -> ()  [unwired: 3 in, 1 out]
      }
      n67 = call <vilib>:"Linear Fit.vi"("Y"=w157, "X"=w193, "method"=w198) -> ("slope"=w197:dbl)  [unwired: 8 in, 4 out]
      n68 = call "Convert to Dynamic Data"("Array"=w193) -> ("Dynamic Data Type"=w200:dynamicdata)  [unwired: 3 in]
      n69 = call "Convert to Dynamic Data2"("Array"=w157) -> ("Dynamic Data Type"=w199:dynamicdata)  [unwired: 3 in]
      n70 = call "Open Circuit Voltage & Short Circuit Current.vi"("current"=w157, "voltage"=w193) -> ("open circuit voltage"=w189:dbl, "short circuit current"=w190:dbl, "Current (Amps) vs Voltage (Volts)"=w195:cluster{"voltage":dbl[], "current":dbl[]})  [unwired: 7 out]
      "Voc (Volts)" <- w189
      "Isc (Amps)" <- w190
      n71 = Reciprocal(x=w197) -> (1/x=w181:dbl)
      "Fit linear R (Ohms)" <- w181
      n72 = call "Build XY Graph"("Reset"=TRUE, "Y Input"=w199, "X Input"=w200) -> ("XY Graph"=→"Curva I(V)":cluster{"Y":dbl[], "Y":dbl[]}[])  [unwired: 7 in, 1 out]
      n73 = Format Value(value (0)=w181) -> (output string=w166:string)  [unwired: 2 in]
      n74 = call "Maximum Power.vi"("Current (Amps) vs Voltage (Volts)"=w195) -> ("max power"=w187:dbl, "Power (Watts) vs Voltage (Volts)"=w194:cluster{"voltage":dbl[], dbl[]}, "current at max power"=w186:dbl, "voltage at max power"=w185:dbl)  [unwired: 7 out]
      "Imp (Amps)" <- w186
      "Vmp (Volts)" <- w185
      "Pmax (Watts)" <- w187
      n75 = Format Value(value (0)=w190) -> (output string=w177:string)  [unwired: 2 in]
      n76 = Format Value(value (0)=w189) -> (output string=w176:string)  [unwired: 2 in]
      n77 = call "R@Isc and R@Voc.vi"("percentage"=sgl 0.075, "Current (Amps) vs Voltage (Volts)"=w195) -> ("Rseries"=w182:dbl, "Rshunt"=w183:dbl)  [unwired: 8 out]
      "Rshunt (Ohms)" <- w183
      "Rseries (Ohms)" <- w182
      n78 = Build Array(w195, w194) -> (w165:cluster{"voltage":dbl[], "current":dbl[]}[])
      n79 = call "Fill Factor.vi"("Current at Short Circuit"=w190, "Voltage at Open Circuit"=w189, "Voltage at Max Power"=w185, "Current at Max Power"=w186) -> ("fill factor"=w184:dbl)  [unwired: 7 out]
      "Fill Factor" <- w184
      n80 = call "Efficiencycode.vi"("Maximum Power"=w187, "Irradiance"=w180, "Area"="Área total das células (m²)") -> ("Efficiency"=w188:dbl)  [unwired: 1 in, 7 out]
      "Efficiency (%)" <- w188
      n81 = Format Value(value (0)="Área total das células (m²)") -> (output string=w167:string)  [unwired: 2 in]
      n82 = Format Value(value (0)=w180) -> (output string=w168:string)  [unwired: 2 in]
      n83 = Format Value(value (0)=w187) -> (output string=w170:string)  [unwired: 2 in]
      n84 = Format Value(value (0)=w186) -> (output string=w171:string)  [unwired: 2 in]
      n85 = Format Value(value (0)=w185) -> (output string=w172:string)  [unwired: 2 in]
      n86 = Format Value(value (0)=w183) -> (output string=w174:string)  [unwired: 2 in]
      n87 = Format Value(value (0)=w182) -> (output string=w175:string)  [unwired: 2 in]
      n88 = Format Value(value (0)=w188) -> (output string=w169:string)  [unwired: 2 in]
      n89 = Format Value(value (0)=w184) -> (output string=w173:string)  [unwired: 2 in]
      n90 = Format Value(value (0)=w163) -> (output string=w179:string)  [unwired: 2 in]
      n91 = Format Value(format string="%#g", value (0)="Nº de células") -> (output string=w178:string)  [unwired: 1 in]
    }
    frame #3 {
      n92 = call <instrlib>:"Input Control.vi"("Enable Input Terminals (F: Off)"=FALSE ("Enable Output (T: Enable)"), "VISA resource name"=w235) -> ("error out"=w233:errorcluster, "VISA resource name out"=w234:refnum<visa-resource-name>)  [unwired: 8 in]
      n93 = call <instrlib>:"Close.vi"("error in (no error)"=w233, "VISA resource name"=w234) -> ()  [unwired: 9 in, 1 out]
    }
    frame #4 {
      (unwired) TRUE ("append on new line? (F)")
      (unwired) TRUE ("append on new line? (F)")
      n94 = call <vilib>:"New Report.vi"("report type"=T4."HTML") -> ("report out"=w254:refnum<class "NI_report.lvclass">, "error out"=w255:errorcluster)  [unwired: 13 in]
      n95 = call-dynamic "Set Report Header Text.vi"("report in"=w254, "center header text"="Relatório de medidas", "error in (no error)"=w255) -> ("report out"=w257:refnum<class "NI_report.lvclass">, "error out"=w258:errorcluster)  [unwired: 11 in]
      n96 = call-poly <vilib>:"Append Report Text.vi"("report in"=w257, "text"="Medidas realizadas no dia ", "append on new line? (F)"=TRUE, "error in (no error)"=w258) -> ("report out"=w261:refnum<class "NI_report.lvclass">, "error out"=w262:errorcluster)  [unwired: 8 in, 2 out]
      n97 = Get Date/Time String(want seconds? (F)=TRUE) -> (date string=w263:string, time string=w269:string)  [unwired: 2 in]
      n98 = call-poly <vilib>:"Append Report Text.vi"("report in"=w261, "text"=w263, "error in (no error)"=w262) -> ("report out"=w264:refnum<class "NI_report.lvclass">, "error out"=w265:errorcluster)  [unwired: 9 in, 2 out]
      n99 = call-poly <vilib>:"Append Report Text.vi"("report in"=w264, "text"=" às ", "error in (no error)"=w265) -> ("report out"=w267:refnum<class "NI_report.lvclass">, "error out"=w268:errorcluster)  [unwired: 9 in, 2 out]
      n100 = call-poly <vilib>:"Append Report Text.vi"("report in"=w267, "text"=w269, "error in (no error)"=w268) -> ("report out"=w271:refnum<class "NI_report.lvclass">, "error out"=w272:errorcluster)  [unwired: 9 in, 2 out]
      n101 = call-dynamic "Set Report Font.vi"("report in"=w271, "text options"=T3 {"Italic"=enum."Italic Unchanged", "Strike Through"=enum."Strike Through Unchanged", "Underline"=enum."Underline Unchanged", "Bold"=enum."Bold On"}, "error in (no error)"=w272) -> ("report out"=w274:refnum<class "NI_report.lvclass">, "error out"=w276:errorcluster)  [unwired: 10 in, 1 out]
      n102 = call-dynamic "New Report Line.vi"("report in"=w274, "number of lines (1)"=2, "error in (no error)"=w276) -> ("report out"=w275:refnum<class "NI_report.lvclass">, "error out"=w277:errorcluster)  [unwired: 11 in]
      n103 = call-poly <vilib>:"Append Report Text.vi"("report in"=w275, "text"="Parâmetros utilizados:", "error in (no error)"=w277) -> ("report out"=w280:refnum<class "NI_report.lvclass">, "error out"=w281:errorcluster)  [unwired: 9 in, 2 out]
      n104 = call-dynamic "Set Report Font.vi"("report in"=w280, "text options"=T3 {"Italic"=enum."Italic Unchanged", "Strike Through"=enum."Strike Through Unchanged", "Underline"=enum."Underline Unchanged", "Bold"=enum."Bold Off"}, "error in (no error)"=w281) -> ("report out"=w283:refnum<class "NI_report.lvclass">, "error out"=w284:errorcluster)  [unwired: 10 in, 1 out]
      n105 = call-poly <vilib>:"Append Report Text.vi"("report in"=w283, "text"="Nº de células: ", "append on new line? (F)"=TRUE, "error in (no error)"=w284) -> ("report out"=w286:refnum<class "NI_report.lvclass">, "error out"=w287:errorcluster)  [unwired: 8 in, 2 out]
      n106 = call-poly <vilib>:"Append Report Text.vi"("report in"=w286, "text"=w240, "error in (no error)"=w287) -> ("report out"=w289:refnum<class "NI_report.lvclass">, "error out"=w290:errorcluster)  [unwired: 9 in, 2 out]
      n107 = call-poly <vilib>:"Append Report Text.vi"("report in"=w289, "text"="Área (m²): ", "append on new line? (F)"=TRUE, "error in (no error)"=w290) -> ("report out"=w293:refnum<class "NI_report.lvclass">, "error out"=w294:errorcluster)  [unwired: 8 in, 2 out]
      n108 = call-poly <vilib>:"Append Report Text.vi"("report in"=w293, "format string (%.3f)"="%8e", "text"=w252, "error in (no error)"=w294) -> ("report out"=w295:refnum<class "NI_report.lvclass">, "error out"=w296:errorcluster)  [unwired: 8 in, 2 out]
      n109 = call-poly <vilib>:"Append Report Text.vi"("report in"=w295, "text"="Luminosidade (W/m²): ", "append on new line? (F)"=TRUE, "error in (no error)"=w296) -> ("report out"=w299:refnum<class "NI_report.lvclass">, "error out"=w300:errorcluster)  [unwired: 8 in, 2 out]
      n110 = call-poly <vilib>:"Append Report Text.vi"("report in"=w299, "text"=w251, "error in (no error)"=w300) -> ("report out"=w365:refnum<class "NI_report.lvclass">, "error out"=w366:errorcluster)  [unwired: 9 in, 2 out]
      n111 = call-poly <vilib>:"Append Report Text.vi"("report in"=w365, "text"="Temperatura (ºC): ", "append on new line? (F)"=TRUE, "error in (no error)"=w366) -> ("report out"=w369:refnum<class "NI_report.lvclass">, "error out"=w370:errorcluster)  [unwired: 8 in, 2 out]
      n112 = call-poly <vilib>:"Append Report Text.vi"("report in"=w369, "text"=w239, "error in (no error)"=w370) -> ("report out"=w390:refnum<class "NI_report.lvclass">, "error out"=w391:errorcluster)  [unwired: 9 in, 2 out]
      n113 = call-dynamic "New Report Line.vi"("report in"=w390, "number of lines (1)"=2, "error in (no error)"=w391) -> ("report out"=w302:refnum<class "NI_report.lvclass">, "error out"=w303:errorcluster)  [unwired: 11 in]
      n114 = call-dynamic "Set Report Font.vi"("report in"=w302, "text options"=T3 {"Italic"=enum."Italic Unchanged", "Strike Through"=enum."Strike Through Unchanged", "Underline"=enum."Underline Unchanged", "Bold"=enum."Bold On"}, "error in (no error)"=w303) -> ("report out"=w305:refnum<class "NI_report.lvclass">, "error out"=w306:errorcluster)  [unwired: 10 in, 1 out]
      n115 = call-poly <vilib>:"Append Report Text.vi"("report in"=w305, "text"="Resultados obtidos:", "error in (no error)"=w306) -> ("report out"=w308:refnum<class "NI_report.lvclass">, "error out"=w309:errorcluster)  [unwired: 9 in, 2 out]
      n116 = call-dynamic "Set Report Font.vi"("report in"=w308, "text options"=T3 {"Italic"=enum."Italic Unchanged", "Strike Through"=enum."Strike Through Unchanged", "Underline"=enum."Underline Unchanged", "Bold"=enum."Bold Off"}, "error in (no error)"=w309) -> ("report out"=w379:refnum<class "NI_report.lvclass">, "error out"=w380:errorcluster)  [unwired: 10 in, 1 out]
      n117 = control-ref of="Current and Power vs. Voltage"() -> (w237:refnum<vi>)
      n118 = call-dynamic "New Report Line.vi"("report in"=w379, "number of lines (1)"=2, "error in (no error)"=w380) -> ("report out"=w381:refnum<class "NI_report.lvclass">, "error out"=w382:errorcluster)  [unwired: 11 in]
      n119 = call-dynamic "Append Control Image to Report.vi"("report in"=w381, "alignment (default)"=HTML_Report_Image_Alignment."MIDDLE", "ctrl reference"=w237, "error in (no error)"=w382) -> ("report out"=w384:refnum<class "NI_report.lvclass">, "error out"=w385:errorcluster)  [unwired: 8 in, 2 out]
      n120 = call-dynamic "New Report Line.vi"("report in"=w384, "number of lines (1)"=2, "error in (no error)"=w385) -> ("report out"=w386:refnum<class "NI_report.lvclass">, "error out"=w387:errorcluster)  [unwired: 11 in]
      n121 = call-poly <vilib>:"Append Report Text.vi"("report in"=w386, "text"="Isc (A): ", "error in (no error)"=w387) -> ("report out"=w312:refnum<class "NI_report.lvclass">, "error out"=w313:errorcluster)  [unwired: 9 in, 2 out]
      n122 = call-poly <vilib>:"Append Report Text.vi"("report in"=w312, "text"=w241, "error in (no error)"=w313) -> ("report out"=w314:refnum<class "NI_report.lvclass">, "error out"=w315:errorcluster)  [unwired: 9 in, 2 out]
      n123 = call-poly <vilib>:"Append Report Text.vi"("report in"=w314, "text"="Voc (V): ", "append on new line? (F)"=TRUE, "error in (no error)"=w315) -> ("report out"=w318:refnum<class "NI_report.lvclass">, "error out"=w319:errorcluster)  [unwired: 8 in, 2 out]
      n124 = call-poly <vilib>:"Append Report Text.vi"("report in"=w318, "text"=w242, "error in (no error)"=w319) -> ("report out"=w320:refnum<class "NI_report.lvclass">, "error out"=w321:errorcluster)  [unwired: 9 in, 2 out]
      n125 = call-poly <vilib>:"Append Report Text.vi"("report in"=w320, "text"="Eficiência (%): ", "append on new line? (F)"=TRUE, "error in (no error)"=w321) -> ("report out"=w324:refnum<class "NI_report.lvclass">, "error out"=w325:errorcluster)  [unwired: 8 in, 2 out]
      n126 = call-poly <vilib>:"Append Report Text.vi"("report in"=w324, "text"=w250, "error in (no error)"=w325) -> ("report out"=w326:refnum<class "NI_report.lvclass">, "error out"=w327:errorcluster)  [unwired: 9 in, 2 out]
      n127 = call-poly <vilib>:"Append Report Text.vi"("report in"=w326, "text"="Pmax (W): ", "append on new line? (F)"=TRUE, "error in (no error)"=w327) -> ("report out"=w330:refnum<class "NI_report.lvclass">, "error out"=w331:errorcluster)  [unwired: 8 in, 2 out]
      n128 = call-poly <vilib>:"Append Report Text.vi"("report in"=w330, "text"=w249, "error in (no error)"=w331) -> ("report out"=w332:refnum<class "NI_report.lvclass">, "error out"=w333:errorcluster)  [unwired: 9 in, 2 out]
      n129 = call-poly <vilib>:"Append Report Text.vi"("report in"=w332, "text"="Imp (A): ", "append on new line? (F)"=TRUE, "error in (no error)"=w333) -> ("report out"=w336:refnum<class "NI_report.lvclass">, "error out"=w337:errorcluster)  [unwired: 8 in, 2 out]
      n130 = call-poly <vilib>:"Append Report Text.vi"("report in"=w336, "text"=w248, "error in (no error)"=w337) -> ("report out"=w338:refnum<class "NI_report.lvclass">, "error out"=w339:errorcluster)  [unwired: 9 in, 2 out]
      n131 = call-poly <vilib>:"Append Report Text.vi"("report in"=w338, "text"="Vmp (V): ", "append on new line? (F)"=TRUE, "error in (no error)"=w339) -> ("report out"=w342:refnum<class "NI_report.lvclass">, "error out"=w343:errorcluster)  [unwired: 8 in, 2 out]
      n132 = call-poly <vilib>:"Append Report Text.vi"("report in"=w342, "text"=w247, "error in (no error)"=w343) -> ("report out"=w344:refnum<class "NI_report.lvclass">, "error out"=w345:errorcluster)  [unwired: 9 in, 2 out]
      n133 = call-poly <vilib>:"Append Report Text.vi"("report in"=w344, "text"="Fill Factor: ", "append on new line? (F)"=TRUE, "error in (no error)"=w345) -> ("report out"=w348:refnum<class "NI_report.lvclass">, "error out"=w349:errorcluster)  [unwired: 8 in, 2 out]
      n134 = call-poly <vilib>:"Append Report Text.vi"("report in"=w348, "text"=w246, "error in (no error)"=w349) -> ("report out"=w350:refnum<class "NI_report.lvclass">, "error out"=w351:errorcluster)  [unwired: 9 in, 2 out]
      n135 = call-poly <vilib>:"Append Report Text.vi"("report in"=w350, "text"="Rshunt (Ohms): ", "append on new line? (F)"=TRUE, "error in (no error)"=w351) -> ("report out"=w354:refnum<class "NI_report.lvclass">, "error out"=w355:errorcluster)  [unwired: 8 in, 2 out]
      n136 = call-poly <vilib>:"Append Report Text.vi"("report in"=w354, "text"=w244, "error in (no error)"=w355) -> ("report out"=w356:refnum<class "NI_report.lvclass">, "error out"=w357:errorcluster)  [unwired: 9 in, 2 out]
      n137 = call-poly <vilib>:"Append Report Text.vi"("report in"=w356, "text"="Rseries (Ohms): ", "append on new line? (F)"=TRUE, "error in (no error)"=w357) -> ("report out"=w360:refnum<class "NI_report.lvclass">, "error out"=w361:errorcluster)  [unwired: 8 in, 2 out]
      n138 = call-poly <vilib>:"Append Report Text.vi"("report in"=w360, "text"=w243, "error in (no error)"=w361) -> ("report out"=w375:refnum<class "NI_report.lvclass">, "error out"=w376:errorcluster)  [unwired: 9 in, 2 out]
      n139 = call-poly <vilib>:"Append Report Text.vi"("report in"=w375, "text"="Fit linear R (Ohms): ", "append on new line? (F)"=TRUE, "error in (no error)"=w376) -> ("report out"=w371:refnum<class "NI_report.lvclass">, "error out"=w372:errorcluster)  [unwired: 8 in, 2 out]
      n140 = call-poly <vilib>:"Append Report Text.vi"("report in"=w371, "text"=w245, "error in (no error)"=w372) -> ("report out"=w377:refnum<class "NI_report.lvclass">, "error out"=w378:errorcluster)  [unwired: 9 in, 2 out]
      n141 = call-dynamic "Save Report to File.vi"("report in"=w377, "report file path"="Salvar relatório em", "error in (no error)"=w378) -> ("report out"=w363:refnum<class "NI_report.lvclass">, "error out"=w364:errorcluster)  [unwired: 11 in]
      n142 = call-dynamic "Dispose Report.vi"("report in"=w363, "error in (no error)"=w364) -> ()  [unwired: 13 in, 1 out]
      "Current and Power vs. Voltage" <- w238
    }
  }
